vi "Get LeafNodes[].vi"(8 "error in (no error)":errorcluster caption="错误输入（无错误）", 11 "PanelRootNode 输入":refnum<class "PanelRootNode.lvclass"> caption="DNL_LabVIEW Object in") -> (0 "error out":errorcluster caption="错误输出", 2 "LeafNodes[]":refnum<data-value>[](array[refnum]), 3 "PanelRootNode 输出":refnum<class "PanelRootNode.lvclass"> caption="DNL_LabVIEW Object out")   [LabVIEW 2016, in "PanelRootNode.lvclass"]
uses:
  PanelRootNode.lvclass
  PanelObject/PanelObject.lvclass
  PanelRootNode.lvclass/PanelRootNode.ctl
  PanelDataNode/PanelDataNode.lvclass
  C:/Users/CL/Desktop/ZcDAQprj0811/ZcDAQprj/Modules/DAQ-Display/PanelSplitToolkit/PanelObject/PanelObject.lvclass
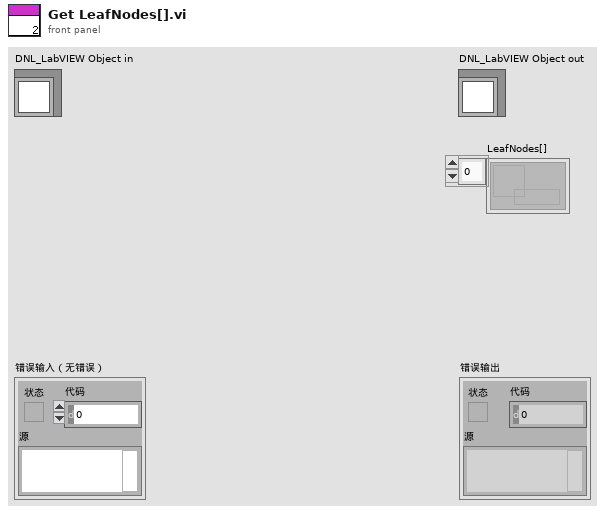
[diagram p1: front panel]
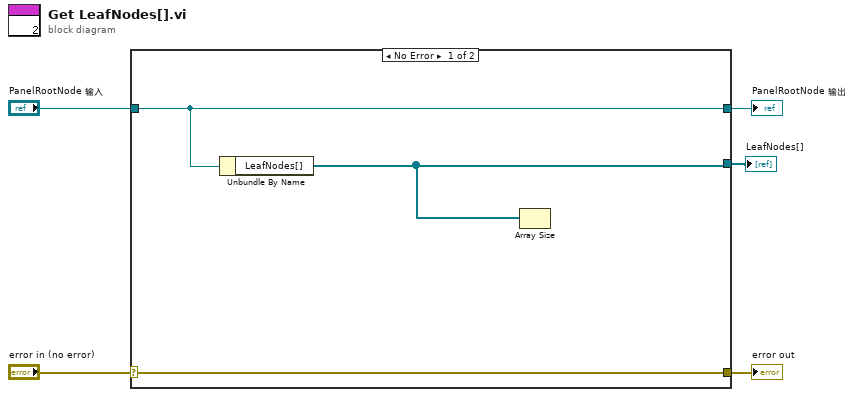
[diagram p0: block diagram]
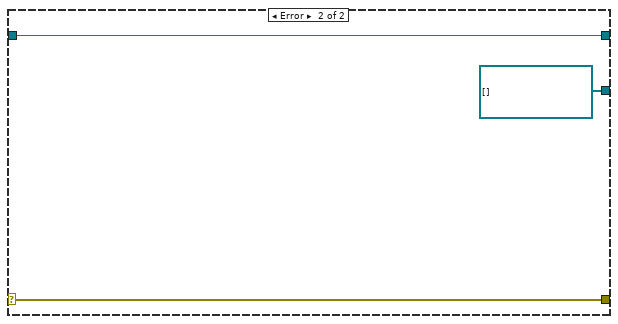
[diagram p2: hidden frame]
diagram:
  n1 = case shown="No Error" "error in (no error)" {
    selector: "error in (no error)" -> [w7 w11]
    tunnel: [w7 w11] -> w4
    tunnel: [w8 w10] -> w2
    tunnel: "PanelRootNode 输入" -> [w8 w10]
    tunnel: [w6 refnum<data-value>[] [] ("LeafNodes[]")] -> w1
    frame No Error {
      n2 = Unbundle By Name(w8) -> ("LeafNodes[]"=w6:refnum<data-value>[])
      n3 = Array Size(array=w6) -> ()  [unwired: 1 out]
    }
    frame Error {
    }
  }
  "error out" <- w4
  "PanelRootNode 输出" <- w2
  "LeafNodes[]" <- w1
